vi "SPARK Get Alt Ext Encoder Status.vi"   [LabVIEW 2023]
doc: "Get the periodic status from the alternate or external encoder encoder connected to the data port of the SPARK."
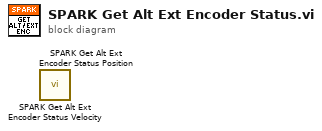
[diagram p0: block diagram]
diagram:
  n1 = call "SPARK Get Alt Ext Encoder Status Velocity.vi"() -> ()  [unwired: 8 in, 4 out]
  n2 = call "SPARK Get Alt Ext Encoder Status Position.vi"() -> ()  [unwired: 8 in, 4 out]
